vi "Subvi FileName Valid.vi"(1 "InFileName":string) -> (0 "Success":bool)   [LabVIEW 2012]
doc: "This Vi takes a filename and parses to make sure that only alphanumeric, space and underscore characters are present. Returns boolean if successful."
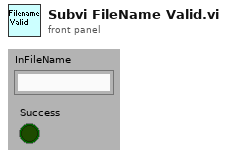
[diagram p1: front panel]
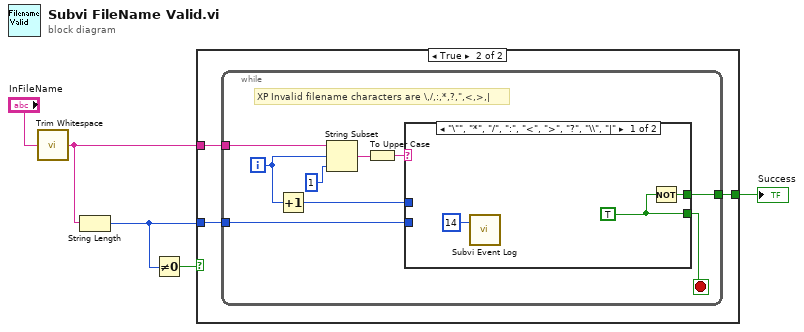
[diagram p0: block diagram]
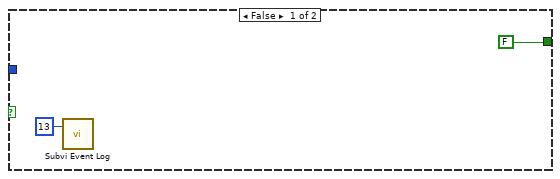
[diagram p2: hidden frame]
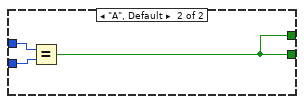
[diagram p3: hidden frame]
diagram:
  n1 = call <vilib>:"Trim Whitespace.vi"("string"="InFileName") -> ("trimmed string"=w4:string)  [unwired: 1 in]
  n2 = String Length(string=w4) -> (length=w2:i32)
  n3 = Not Equal To 0?(x=w2) -> (x != 0?=w1:bool)
  n4 = case shown="True" w1 {
    tunnel: w4 -> [_ w10]
    tunnel: w2 -> [_ w9]
    tunnel: [FALSE w8] -> w3
    frame False {
      n5 = call "Subvi Event Log.vi"("EventNum"=u32 13) -> ()  [unwired: 1 in]
    }
    frame True {
      n6 = while {
        tunnel: w10 -> [w16]
        tunnel: w9 -> [w14]
        tunnel: [w12] -> w8
        i -> [w15]
        stop <- w11 stop-if-true
        # "XP Invalid filename characters are \\,/,:,*,?,\",<,>,|"
        n7 = Increment(x=w15) -> (x+1=w13:i32)
        n8 = String Subset(string=w16, offset (0)=w15, length (rest)=1 ("length (rest)")) -> (substring=w18:string)
        n9 = To Upper Case(1:w18) -> (0:w17:string)
        n10 = case shown="\"\\\"\", \"*\", \"/\", \":\", \"<\", \">\", \"?\", \"\\\\\", \"|\"" w17 {
          tunnel: [w20 w23] -> w11
          tunnel: w14 -> [_ w25]
          tunnel: w13 -> [_ w24]
          tunnel: [w22 w23] -> w12
          frame "\"", "*", "/", ":", "<", ">", "?", "\\", "|" {
            w20 = TRUE
            n11 = call "Subvi Event Log.vi"("EventNum"=u32 14) -> ()  [unwired: 1 in]
            n12 = Not(x=w20) -> (.not. x?=w22:bool)
          }
          frame "A", Default {
            n13 = Equal?(x=w24, y=w25) -> (x = y?=w23:bool)
          }
        }
      }
    }
  }
  "Success" <- w3
